vi "Gen - Popup Two Button.vi"(6 "Type":enum16{"Error", "Info"}(ring)=enum."Info", 8 "Error in":errorcluster, 9 "Button text":string[](array[string])=["YES", "NO"], 10 "Message in":string, 11 "Header":string) -> (0 "Error out":errorcluster, 3 "Yes?":bool)   [LabVIEW 2020]
uses:
  Control/State - eFGV.ctl
panel:
  out "Type Error":bool
  in  "No":bool
  in  "Yes":bool
  in  "Cancel":bool
  out "Type Info":bool
  in  "OK":bool
  out "Header out":string
  in  "Exit":bool
  out "Message":string
  in  "Auto Close?":bool
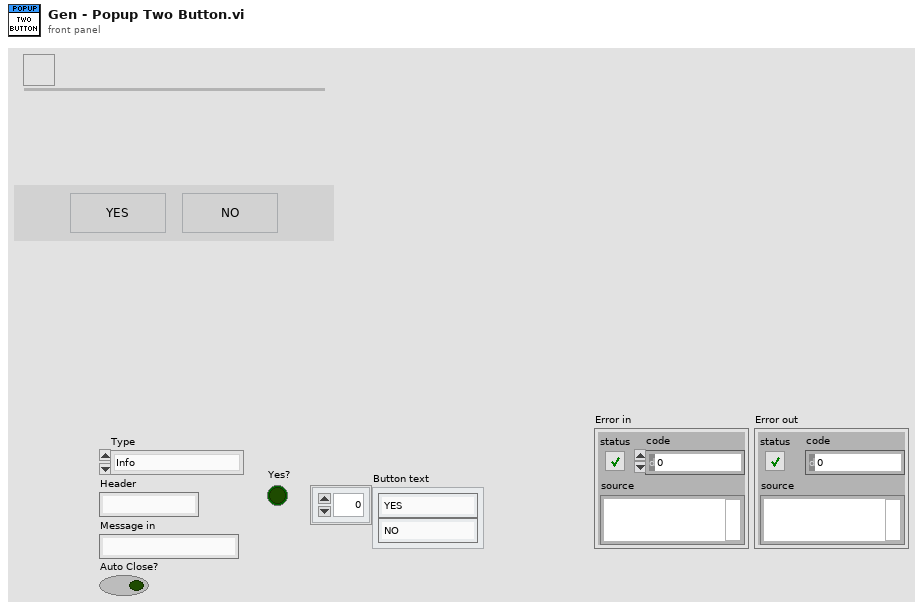
[diagram p1: front panel]
types:
  T1 = typedef "State - eFGV.ctl" = enum16{"Init", "Read", "Write", "Exit"}
  T2 = enum32{"Invalid", "Default", "Floating", "Floating/Auto-Hide", "Modal"}
  T3 = enum8{"Enabled", "Disabled", "Disabled and Grayed Out"}
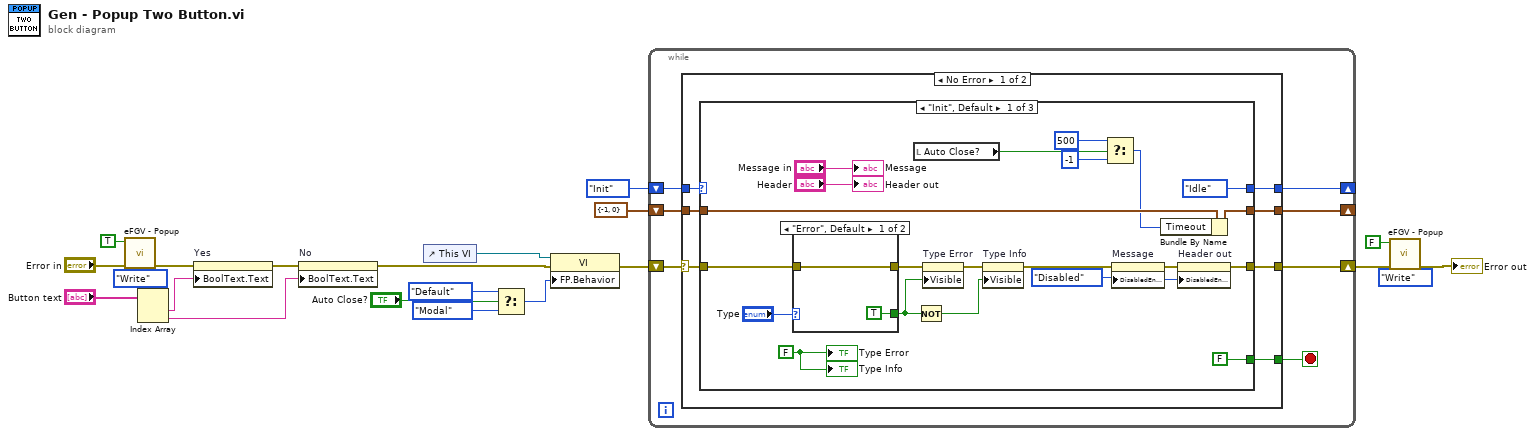
[diagram p0: block diagram]
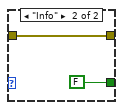
[diagram p2: hidden frame]
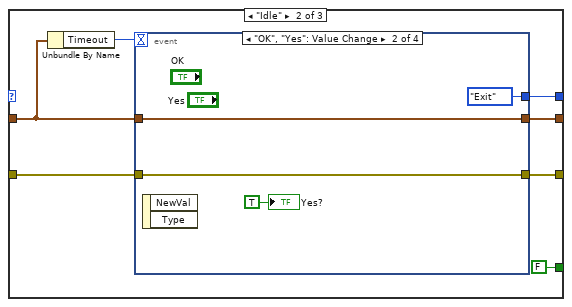
[diagram p3: hidden frame]
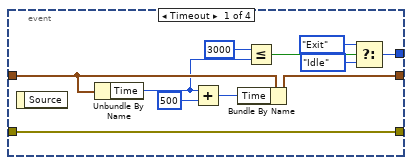
[diagram p4: hidden frame]
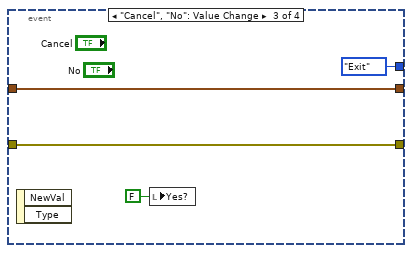
[diagram p5: hidden frame]
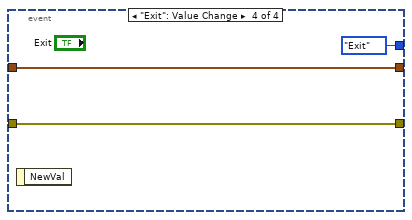
[diagram p6: hidden frame]
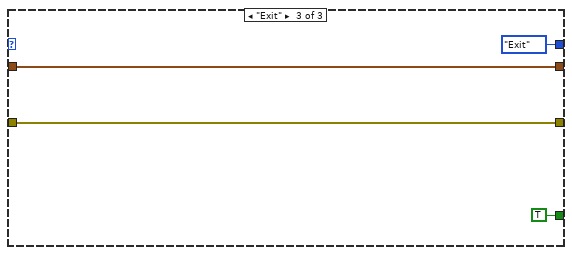
[diagram p7: hidden frame]
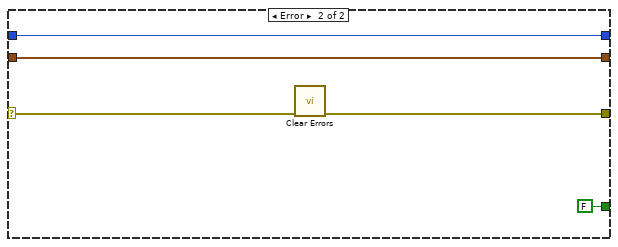
[diagram p8: hidden frame]
diagram:
  n1 = call "eFGV - Popup.vi"("Action"=State_-_eFGV."Write", "Error In"="Error in", "Popup"=TRUE) -> ("Error Out"=w8:errorcluster)  [unwired: 6 in, 2 out]
  n2 = Index Array(array="Button text") -> (element #1=w10:string, element #2=w9:string)  [unwired: 2 in]
  n3 = property on="Yes" class="Bool"(error in=w8, "BoolText.Text"=w10) -> (error out=w13:errorcluster)  [unwired: 1 in, 1 out]
  n4 = property on="No" class="Bool"(error in=w13, "BoolText.Text"=w9) -> (error out=w12:errorcluster)  [unwired: 1 in, 1 out]
  n5 = control-ref of="This VI"() -> (w19:refnum<vi>)
  n6 = Select(t=T2."Default" ("Front Panel Window:Behavior"), s="Auto Close?", f=T2."Modal") -> (s? t:f=w15:T2)
  n7 = property class="VI"(reference=w19, error in=w12, "FP.Behavior"=w15) -> (error out=w18:errorcluster)  [unwired: 1 out]
  n8 = while {
    shift-right: [w26] -> _
    shift-left: enum16{"Init", "Idle", "Exit"}."Init" -> [w27]
    shift-right: [w25] -> w4
    shift-left: w18 -> [w28]
    shift-right: [w22] -> _
    shift-left: cluster{"Timeout":i32, "Time":i32} {"Timeout"=-1, "Time"=0} -> [w23]
    stop <- w24 stop-if-true
    n9 = case shown="No Error" w28 {
      selector: w28 -> [w32 w97]
      tunnel: w27 -> [w35 w98]
      tunnel: [w34 w98] -> w26
      tunnel: [w33 w95] -> w25
      tunnel: [w31 FALSE] -> w24
      tunnel: w23 -> [w30 w94]
      tunnel: [w29 w94] -> w22
      frame No Error {
        n10 = case shown="\"Init\", Default" w35 {
          tunnel: [enum16{"Init", "Idle", "Exit"}."Idle" w67 enum16{"Init", "Idle", "Exit"}."Exit"] -> w34
          tunnel: [w41 w66 w93] -> w33
          tunnel: w32 -> [w48 w65 w93]
          tunnel: [FALSE FALSE TRUE] -> w31
          tunnel: w30 -> [w52 w62 w90]
          tunnel: [w51 w63 w90] -> w29
          frame "Init", Default {
            w44 = T3."Disabled" ("Disabled")
            w36 = FALSE ("Type Error")
            n11 = case shown="\"Error\", Default" "Type" {
              tunnel: [w57 w60] -> w49
              tunnel: w48 -> [w57 w60]
              tunnel: [TRUE FALSE] -> w46
              frame "Error", Default {
              }
              frame "Info" {
              }
            }
            n12 = local read "Auto Close?"() -> (w37:bool)
            n13 = Not(x=w46) -> (.not. x?=w45:bool)
            n14 = property on="Type Error" class="Bool"(error in=w49, "Visible"=w46) -> (error out=w50:errorcluster)  [unwired: 1 in, 1 out]
            n15 = property on="Type Info" class="Bool (strict)"(error in=w50, "Visible"=w45) -> (error out=w42:errorcluster)  [unwired: 1 in, 1 out]
            n16 = Select(t=500 ("Timeout"), s=w37, f=-1 ("Timeout")) -> (s? t:f=w39:i32)
            n17 = property on="Message" class="Str"(error in=w42, "DisabledEnum"=w44) -> (error out=w43:errorcluster)  [unwired: 1 in, 1 out]
            n18 = Bundle By Name(cluster=w52, "Timeout"=w39) -> (w51:cluster{"Timeout":i32, "Time":i32})
            n19 = property on="Header out" class="Str"(error in=w43, "DisabledEnum"=w44) -> (error out=w41:errorcluster)  [unwired: 1 in, 1 out]
            "Message" <- "Message in"
            "Header out" <- "Header"
            "Type Info" <- w36
            "Type Error" <- w36
          }
          frame "Idle" {
            n20 = Unbundle By Name(w62) -> ("Timeout"=w61:i32)
            n21 = event shown="[1] \"OK\", \"Yes\": Value Change" {
              selector: _ -> [_ _ _ _]
              dyn-events: _ -> [_ _ _ _]
              timeout: w61 -> [_ _ _ _]
              tunnel: [w70 enum16{"Init", "Idle", "Exit"}."Exit" enum16{"Init", "Idle", "Exit"}."Exit" enum16{"Init", "Idle", "Exit"}."Exit"] -> w67
              tunnel: [w78 w80 w84 w87] -> w66
              tunnel: w65 -> [w78 w80 w84 w87]
              tunnel: [w76 w81 w85 w88] -> w63
              tunnel: w62 -> [w77 w81 w85 w88]
              event Timeout {
                n22 = event-data() -> ()  [unwired: 1 in, 1 out]
                n23 = Unbundle By Name(w77) -> ("Time"=w73:i32)
                n24 = Add(x=w73, y=500) -> (x+y=w75:i32)
                n25 = Bundle By Name(cluster=w77, "Time"=w75) -> (w76:cluster{"Timeout":i32, "Time":i32})
                n26 = Less Or Equal?(x=3000, y=w73) -> (x <= y?=w71:bool)
                n27 = Select(t=enum16{"Init", "Idle", "Exit"}."Exit", s=w71, f=enum16{"Init", "Idle", "Exit"}."Idle") -> (s? t:f=w70:enum16{"Init", "Idle", "Exit"})
              }
              event "OK", "Yes": Value Change {
                n28 = event-data() -> ()  [unwired: 1 in, 2 out]
                "Yes?" <- TRUE ("Yes?")
              }
              event "Cancel", "No": Value Change {
                n29 = event-data() -> ()  [unwired: 1 in, 2 out]
                n30 = local write "Yes?"(FALSE ("Yes?")) -> ()
              }
              event "Exit": Value Change {
                n31 = event-data() -> ()  [unwired: 1 in, 1 out]
              }
            }
          }
          frame "Exit" {
          }
        }
      }
      frame Error {
        n32 = call <vilib>:"Clear Errors.vi"("error in (no error)"=w97) -> ("error out"=w95:errorcluster)  [unwired: 5 in, 1 out]
      }
    }
  }
  n33 = call "eFGV - Popup.vi"("Action"=State_-_eFGV."Write", "Error In"=w4, "Popup"=FALSE) -> ("Error Out"=→"Error out":errorcluster)  [unwired: 6 in, 2 out]
